vi "SetDigitalOut.vi"(8 "Error in":errorcluster, 11 "DevicesAndSignals":T1) -> (0 "Error out":errorcluster, 3 "DevicesAndSignals":T1)   [LabVIEW 2016]
doc: "Use this VI to set selected digital out signals to high or low."
panel:
  in  "SetToLow":bool
  in  "SetToHigh":bool
  in  "Signals":i32(listbox)
  in  "stop":bool caption="Stopp"
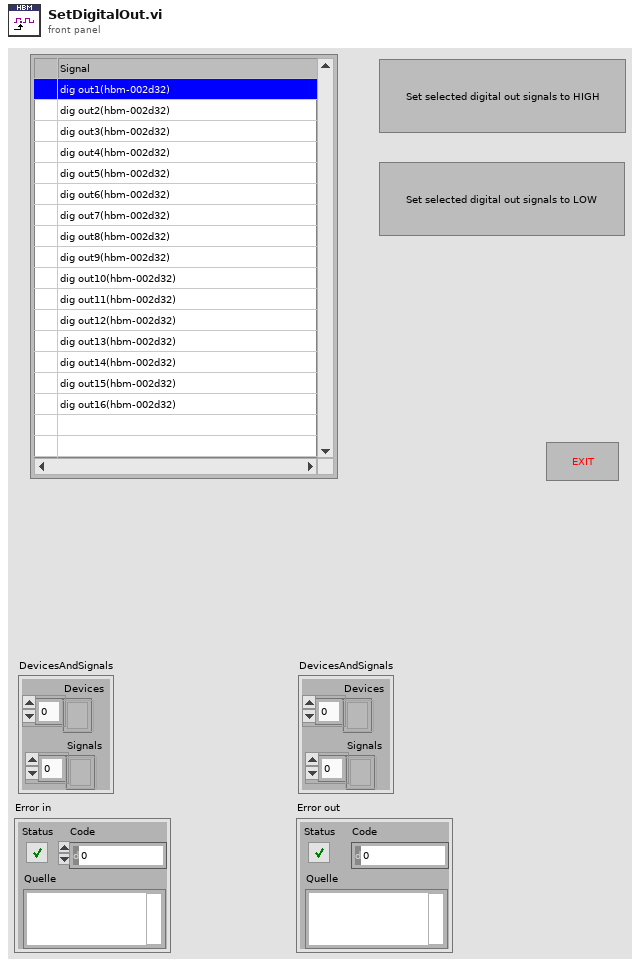
[diagram p1: front panel]
types:
  T1 = cluster{"Devices":refnum<k24>[], "Signals":refnum<k24>[]}
  T2 = typedef "LVPoint32TypeDef.ctl" = cluster{"Horizontal":i32, "Vertical":i32}
  T3 = typedef "LVRowAndColumnTypeDef.ctl" = cluster{"Row":i32, "Column":i32}
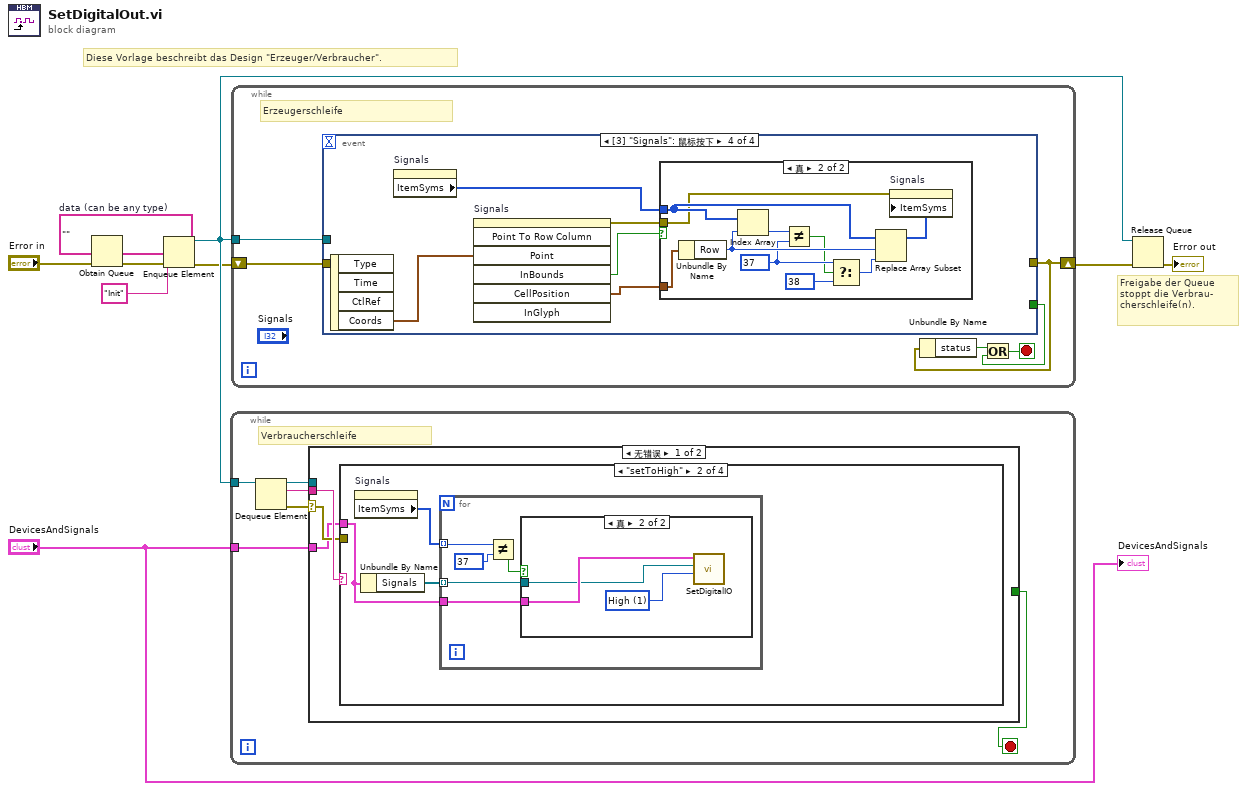
[diagram p0: block diagram]
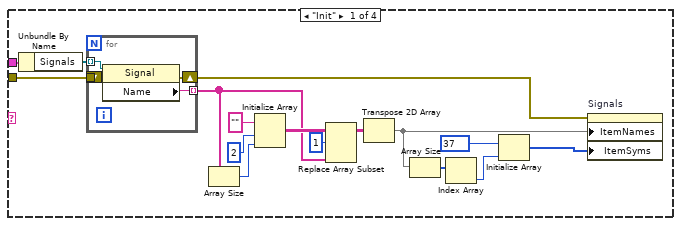
[diagram p2: hidden frame]
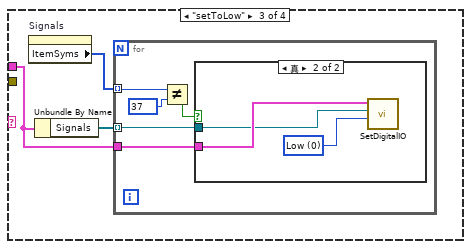
[diagram p4: hidden frame]
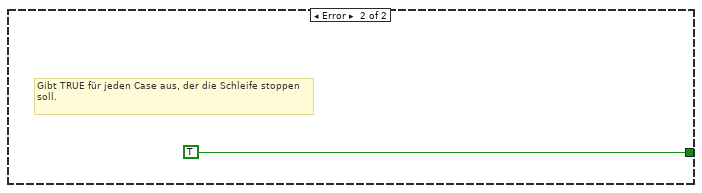
[diagram p7: hidden frame]
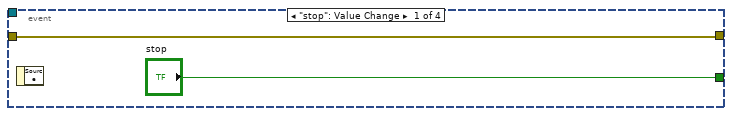
[diagram p8: hidden frame]
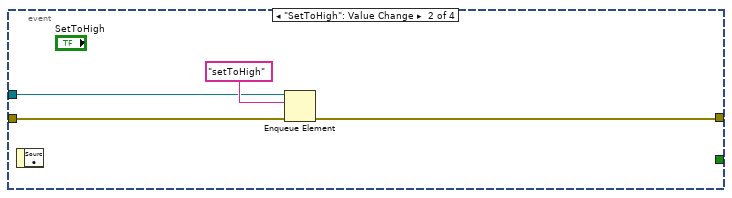
[diagram p9: hidden frame]
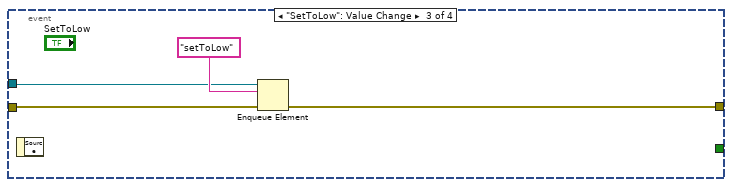
[diagram p10: hidden frame]
diagram:
  w9 = ""  # data (can be any type)
  # "Freigabe der Queue stoppt die Verbrau-\ncherschleife(n)."
  # "Diese Vorlage beschreibt das Design \"Erzeuger/Verbraucher\"."
  n1 = Obtain Queue(element data type=w9, error in (no error)="Error in") -> (queue out=w8:refnum<queue>, error out=w7:errorcluster)  [unwired: 3 in, 1 out]
  n2 = Enqueue Element(queue=w8, element="Init" ("Element"), error in (no error)=w7) -> (queue out=w6:refnum<queue>, error out=w5:errorcluster)  [unwired: 1 in, 1 out]
  n3 = while {
    tunnel: w6 -> [w16]
    tunnel: "DevicesAndSignals" -> [w12]
    stop <- w11 stop-if-true
    # "Verbraucherschleife"
    n4 = Dequeue Element(queue=w16) -> (queue out=w14:refnum<queue>, element=w15:string, error out=w13:errorcluster)  [unwired: 2 in, 1 out]
    n5 = case shown="无错误" w13 {
      selector: w13 -> [w18 _]
      tunnel: w15 -> [w19 _]
      tunnel: [_ TRUE] -> w11
      tunnel: w14 -> [_ _]
      tunnel: w12 -> [w17 _]
      frame No Error {
        n6 = case shown="\"setToHigh\"" w19 {
          tunnel: w18 -> [w24 _ _ _]
          tunnel: w17 -> [w23 w40 w51 _]
          frame "Init" {
            n7 = Unbundle By Name(w23) -> ("Signals"=w35:refnum<k24>[])
            n8 = for {
              tunnel: [w39] -> w25 mode=indexing
              tunnel: w24 -> [w38]
              tunnel: w35 -> [w37] mode=indexing
              shift-right: [w36] -> w22
              shift-left: _ -> [_]
              n9 = property on="Eigenschaftsknoten" class="Signal"(reference=w37, error in=w38) -> (error out=w36:errorcluster, "Name"=w39:string)  [unwired: 1 out]
            }
            n10 = Array Size(array=w25) -> (size(s)=w29:i32)
            n11 = Initialize Array("" ("Element"), 2 ("Dimension"), w29) -> (w33:string[][])
            n12 = Replace Array Subset(array=w33, new element=w25, index (row)=1 ("Index (Zeile)")) -> (w31:string[][])  [unwired: 1 in]
            n13 = Transpose 2D Array(2D array=w31) -> (transposed array=w21:string[][])
            n14 = Array Size(array=w21) -> (size(s)=w28:i32[])
            n15 = Index Array(array=w28) -> (element=w27:i32)  [unwired: 1 in]
            n16 = Initialize Array(37, w27) -> (w20:i32[])
            n17 = property on="Signals" class="MCListbox (严格)"(error in=w22, "ItemNames"=w21, "ItemSyms"=w20) -> ()  [unwired: 1 in, 2 out]
          }
          frame "setToHigh" {
            n18 = property on="Signals" class="MCListbox (严格)"() -> ("ItemSyms"=w42:i32[])  [unwired: 2 in, 2 out]
            n19 = Unbundle By Name(w40) -> ("Signals"=w41:refnum<k24>[])
            n20 = for {
              tunnel: w42 -> [w46] mode=indexing
              tunnel: w41 -> [w43] mode=indexing
              tunnel: w40 -> [w44]
              n21 = Not Equal?(x=w46, y=37) -> (x != y?=w45:bool)
              n22 = case shown="真" w45 {
                tunnel: w44 -> [_ w50]
                tunnel: w43 -> [_ w49]
                frame False {
                }
                frame True {
                  w48 = 1 items=["Low", "High"] ("Value")
                  n23 = call "SetDigitalIO.vi"("Value"=w48, "Signal"=w49, "DevicesAndSignals"=w50) -> ()  [unwired: 7 in, 2 out]
                }
              }
            }
          }
          frame "setToLow" {
            n24 = property on="Signals" class="MCListbox (严格)"() -> ("ItemSyms"=w53:i32[])  [unwired: 2 in, 2 out]
            n25 = Unbundle By Name(w51) -> ("Signals"=w52:refnum<k24>[])
            n26 = for {
              tunnel: w53 -> [w57] mode=indexing
              tunnel: w52 -> [w54] mode=indexing
              tunnel: w51 -> [w55]
              n27 = Not Equal?(x=w57, y=37) -> (x != y?=w56:bool)
              n28 = case shown="真" w56 {
                tunnel: w55 -> [_ w61]
                tunnel: w54 -> [_ w60]
                frame False {
                }
                frame True {
                  w59 = 0 items=["Low", "High"] ("Value")
                  n29 = call "SetDigitalIO.vi"("Value"=w59, "Signal"=w60, "DevicesAndSignals"=w61) -> ()  [unwired: 7 in, 2 out]
                }
              }
            }
          }
          frame Default {
          }
        }
      }
      frame Error {
        # "Gibt TRUE für jeden Case aus, der die Schleife stoppen soll."
      }
    }
  }
  n30 = while {
    shift-right: [w64] -> w10
    shift-left: w5 -> [w67]
    tunnel: w6 -> [w68]
    stop <- w65 stop-if-true
    # "Erzeugerschleife"
    n31 = event shown="[3] \"Signals\": 鼠标按下" {
      selector: _ -> [_ _ _ _]
      dyn-events: _ -> [_ _ _ _]
      timeout: _ -> [_ _ _ _]
      tunnel: w68 -> [_ w73 w77 _]
      tunnel: w67 -> [w69 w72 w76 _]
      tunnel: [w69 w71 w75 _] -> w64
      tunnel: ["stop" _ _ _] -> w66
      event "stop": Value Change {
        n32 = event-data() -> ()  [unwired: 1 in, 1 out]
      }
      event "SetToHigh": Value Change {
        n33 = event-data() -> ()  [unwired: 1 in, 1 out]
        n34 = Enqueue Element(queue=w73, element="setToHigh", error in (no error)=w72) -> (error out=w71:errorcluster)  [unwired: 1 in, 2 out]
      }
      event "SetToLow": Value Change {
        n35 = event-data() -> ()  [unwired: 1 in, 1 out]
        n36 = Enqueue Element(queue=w77, element="setToLow", error in (no error)=w76) -> (error out=w75:errorcluster)  [unwired: 1 in, 2 out]
      }
      event "Signals": Mouse Down {
        n37 = event-data() -> ("Coords"=w80:T2)  [unwired: 1 in, 3 out]
        n38 = property on="Signals" class="MCListbox (严格)"() -> ("ItemSyms"=w82:i32[])  [unwired: 2 in, 2 out]
        n39 = invoke on="Signals" class="MehrSpaltFeld (strikt)" method="Point To Row Column"("Point"=w80) -> (error out=w81:errorcluster, "InBounds"=w79:bool, "CellPosition"=w83:T3)  [unwired: 6 in, 4 out]
        n40 = case shown="真" w79 {
          tunnel: w83 -> [_ w87]
          tunnel: w82 -> [_ w86]
          tunnel: w81 -> [_ w84]
          frame False {
          }
          frame True {
            w89 = 37
            n41 = Unbundle By Name(w87) -> ("Row"=w93:i32)
            n42 = Index Array(array=w86, index=w93) -> (element=w90:i32)
            n43 = Not Equal?(x=w90, y=w89) -> (x != y?=w88:bool)
            n44 = Select(t=w89, s=w88, f=38) -> (s? t:f=w91:i32)
            n45 = Replace Array Subset(array=w86, new element=w91, index=w93) -> (w85:i32[])
            n46 = property on="Signals" class="MCListbox (严格)"(error in=w84, "ItemSyms"=w85) -> ()  [unwired: 1 in, 2 out]
          }
        }
      }
    }
    n47 = Unbundle By Name(w64) -> ("status"=w63:bool)
    n48 = Or(x=w63, y=w66) -> (x .or. y?=w65:bool)
  }
  n49 = Release Queue(queue=w6, error in (no error)=w10) -> (error out=→"Error out":errorcluster)  [unwired: 1 in, 2 out]
  "DevicesAndSignals" <- "DevicesAndSignals"
